vi "GetPrinterName.vi"(0 "error in (no error)":errorcluster caption="错误输入（无错误）") -> (1 "ActivePrinter":string, 2 "PrinterName":string[](array[string]), 3 "error out":errorcluster caption="错误输出")   [LabVIEW 2018]
uses:
  System.Drawing
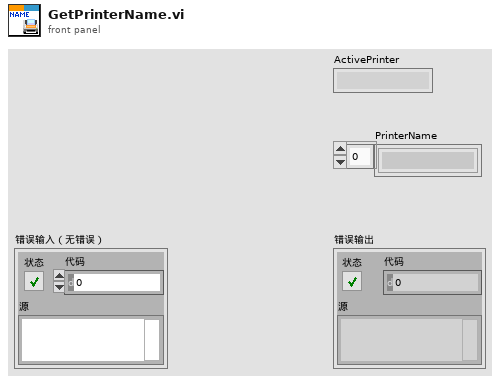
[diagram p1: front panel]
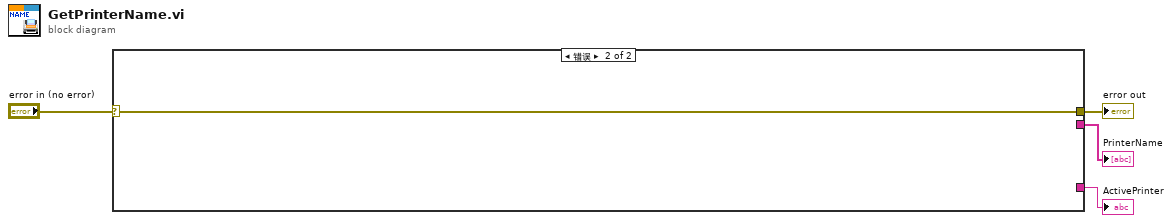
[diagram p0: block diagram]
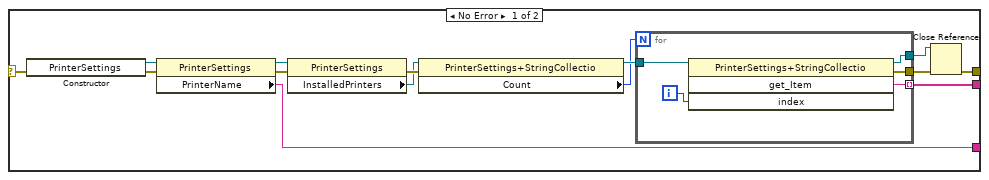
[diagram p2: hidden frame]
diagram:
  n1 = case shown="错误" "error in (no error)" {
    selector: "error in (no error)" -> [w16 w24]
    tunnel: [w5 w24] -> w3
    tunnel: [w15 _] -> w2
    tunnel: [w6 _] -> w1
    frame No Error {
      n2 = constructor class="PrinterSettings"(error in=w16) -> (reference out=w18:refnum<k24>, error out=w17:errorcluster)  [unwired: 2 in, 1 out]
      n3 = property class="PrinterSettings"(reference=w18, error in=w17) -> (reference out=w14:refnum<k24>, error out=w13:errorcluster, "PrinterName"=w15:string)
      n4 = property class="PrinterSettings"(reference=w14, error in=w13) -> (error out=w12:errorcluster, "InstalledPrinters"=w11:refnum<k24>)  [unwired: 1 out]
      n5 = property class="PrinterSettings+StringCollectio"(reference=w11, error in=w12) -> (reference out=w10:refnum<k24>, "Count"=w9:i32)  [unwired: 1 out]
      n6 = for {
        N: w9 -> [_]
        tunnel: w10 -> [w23]
        tunnel: [w21] -> w8
        tunnel: [w20] -> w7
        tunnel: [w19] -> w6 mode=indexing
        i -> [w22]
        n7 = invoke class="PrinterSettings+StringCollectio" method="get_Item"(reference=w23, "index"=w22) -> (reference out=w21:refnum<k24>, error out=w20:errorcluster, "get_Item"=w19:string)  [unwired: 2 in, 1 out]
      }
      n8 = Close Reference(reference=w8, error in (no error)=w7) -> (error out=w5:errorcluster)
    }
    frame Error {
    }
  }
  "error out" <- w3
  "ActivePrinter" <- w2
  "PrinterName" <- w1
